vi "Random_Data Stream Read.vi"(8 "error in":errorcluster, 11 "Call ID in":T2) -> (0 "error out":errorcluster, 1 "Success":bool, 2 "Response Data":T1, 3 "Call ID":T2)   [LabVIEW 2021, in "Stream_client.lvlib"]
uses:
  Stream_client.lvlib
  <vilib>/gRPC/LabVIEW gRPC Library/Shared/grpcId.ctl
  RPC Messages/Acquisition_Stream_Data.ctl
  RPC Messages/Acquisition_Stream_Data_Flat.ctl
  aea5dbbb-03a2-479b-ad95-94da4ee1cea9.vi
  <vilib>/gRPC/LabVIEW gRPC Library/Shared/TranslateGrpcError.vi
  <vilib>/gRPC/LabVIEW gRPC Library/Shared/Wait On Occurrence Wrapper.vi
  <vilib>/gRPC/LabVIEW gRPC Library/Shared/Wait On Occurence.vi
  <vilib>/gRPC/LabVIEW gRPC Library/Server API/Server/Get Server DLL Path.vi
  <vilib>/Utility/error.llb/Error Cluster From Error Code.vi
  <vilib>/Utility/config.llb/Open Config Data.vi
  <vilib>/Utility/config.llb/Write Key.vi
  <vilib>/Utility/config.llb/Write Key (Boolean).vi
  <vilib>/Utility/config.llb/Not A Config Data Refnum.vi
  <vilib>/Utility/config.llb/Read Key.vi
  <vilib>/Utility/config.llb/Read Key (Boolean).vi
  <vilib>/Utility/config.llb/Close Config Data.vi
  <vilib>/gRPC/LabVIEW gRPC Library/grpc-lvsupport-release.lvlib
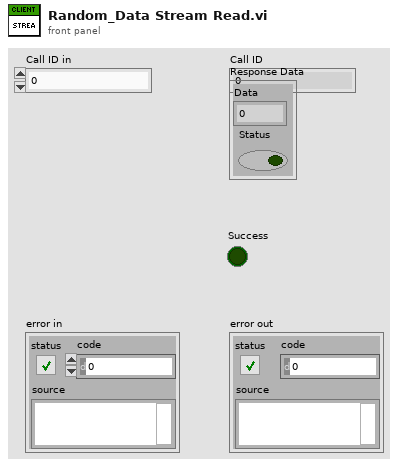
[diagram p1: front panel]
types:
  T1 = typedef "Stream_client.lvlib/Acquisition_Stream_Data.ctl" = cluster{"Data":i32, "Status":bool}
  T2 = typedef "grpc-lvsupport-release.lvlib/grpcId.ctl" = u64
  T3 = typedef "Stream_client.lvlib/Acquisition_Stream_Data_Flat.ctl" = cluster{"Data":i32, "Status":bool}
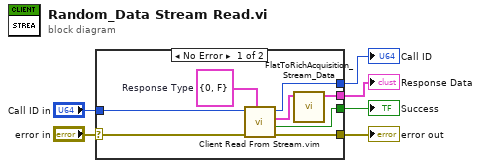
[diagram p0: block diagram]
diagram:
  n1 = case shown="No Error" "error in" {
    selector: "error in" -> [w14 w15]
    tunnel: [w13 w15] -> w5
    tunnel: "Call ID in" -> [w12 w16]
    tunnel: [w10 w16] -> w3
    tunnel: [w7 _] -> w2
    tunnel: [w11 _] -> w1
    frame No Error {
      w9 = T3 {"Data"=0, "Status"=FALSE}  # Response Type
      n2 = call "Client Read From Stream.vim"("Response Type"=w9, "error in"=w14, "Call ID in"=w12) -> ("error out"=w13:errorcluster, "Success"=w11:bool, "Response Data"=w8:T3, "Call ID out"=w10:u64)  [unwired: 5 in]
      n3 = call "FlatToRichAcquisition_Stream_Data.vi"("InputCluster"=w8) -> ("OutputCluster"=w7:T1)  [unwired: 10 in]
    }
    frame Error {
    }
  }
  "error out" <- w5
  "Call ID" <- w3
  "Response Data" <- w2
  "Success" <- w1
